vi "FixPath.vi"(11 "path":string) -> (3 "path":string)   [LabVIEW 2015, in "DiffVI.lvclass"]
uses:
  DiffVI.lvclass
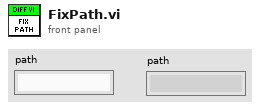
[diagram p1: front panel]
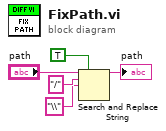
[diagram p0: block diagram]
diagram:
  n1 = Search and Replace String(replace all?=TRUE ("replace all? (F)"), input string="path", search string="/", replace string="\\" ("search string")) -> (result string=→"path":string)  [unwired: 4 in, 3 out]
